vi "Parse Stored String (multibyte).vi"(1 "stored string":string caption="Gespeicherter String") -> (0 "parsed string":string caption="Untersuchter String")   [LabVIEW 2009]
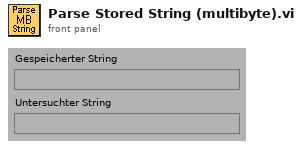
[diagram p1: front panel]
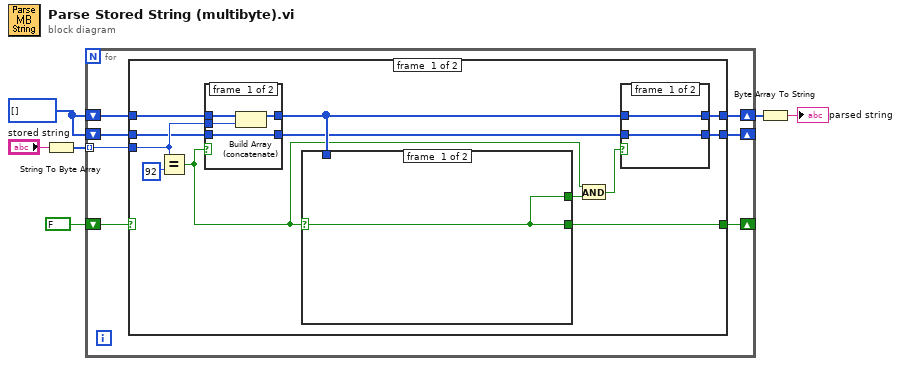
[diagram p0: block diagram]
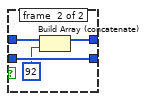
[diagram p2: hidden frame]
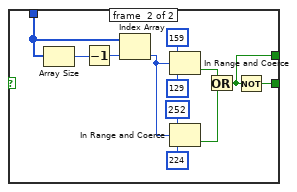
[diagram p3: hidden frame]
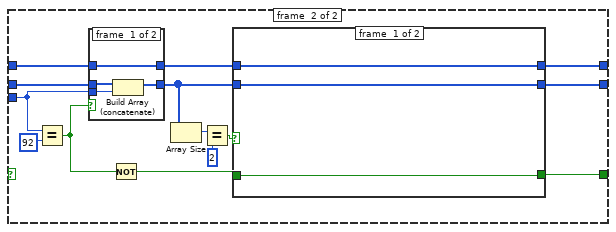
[diagram p5: hidden frame]
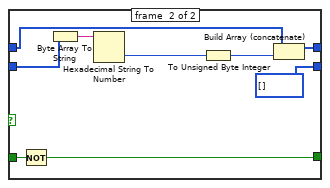
[diagram p6: hidden frame]
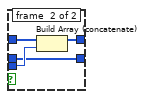
[diagram p7: hidden frame]
diagram:
  w1 = u8[] []
  n1 = String To Byte Array(string="stored string") -> (unsigned byte array=w3:u8[])
  n2 = for {
    tunnel: w3 -> [w9] mode=indexing
    shift-right: [w12] -> w4
    shift-left: w1 -> [w13]
    shift-right: [w10] -> _
    shift-left: FALSE -> [w11]
    shift-right: [w7] -> _
    shift-left: w1 -> [w8]
    n3 = case shown="False" w11 {
      tunnel: w13 -> [w24 w64]
      tunnel: [w17 w54] -> w12
      tunnel: [w21 w52] -> w10
      tunnel: w9 -> [w23 w51]
      tunnel: w8 -> [w22 w61]
      tunnel: [w16 w56] -> w7
      frame #0 {
        n4 = Equal?(x=w23, y=u8 92) -> (x = y?=w14:bool)
        n5 = case shown="False" w14 {
          tunnel: [w47 w50] -> w19
          tunnel: w24 -> [w48 w50]
          tunnel: w23 -> [w46 _]
          tunnel: [w45 w49] -> w18
          tunnel: w22 -> [w45 w49]
          frame #0 {
            n6 = Build Array (concatenate)(w48, w46) -> (w47:u8[])
          }
          frame #1 {
          }
        }
        n7 = case shown="False" w14 {
          selector: w14 -> [w32 _]
          tunnel: w19 -> [_ w42]
          tunnel: [w32 w34] -> w21
          tunnel: [w32 w33] -> w20
          frame #0 {
          }
          frame #1 {
            n8 = Array Size(array=w42) -> (size(s)=w44:i32)
            n9 = Decrement(x=w44) -> (x-1=w43:i32)
            n10 = Index Array(array=w42, index=w43) -> (element=w35:u8)
            n11 = In Range and Coerce(upper limit=u8 159, x=w35, lower limit=u8 129) -> (In Range?=w37:bool)  [unwired: 1 out]
            n12 = In Range and Coerce(upper limit=u8 252, x=w35, lower limit=u8 224) -> (In Range?=w36:bool)  [unwired: 1 out]
            n13 = Or(x=w37, y=w36) -> (x .or. y?=w33:bool)
            n14 = Not(x=w33) -> (.not. x?=w34:bool)
          }
        }
        n15 = And(x=w14, y=w20) -> (x .and. y?=w15:bool)
        n16 = case shown="True" w15 {
          tunnel: [w27 w30] -> w17
          tunnel: w19 -> [w27 w31]
          tunnel: [w26 w29] -> w16
          tunnel: w18 -> [w26 w29]
          frame #0 {
          }
          frame #1 {
            n17 = Build Array (concatenate)(w31, u8 92) -> (w30:u8[])
          }
        }
      }
      frame #1 {
        n18 = Equal?(x=w51, y=u8 92) -> (x = y?=w62:bool)
        n19 = case shown="False" w62 {
          tunnel: w64 -> [w80 w84]
          tunnel: [w80 w83] -> w55
          tunnel: w51 -> [w78 w82]
          tunnel: [w77 w81] -> w57
          tunnel: w61 -> [w79 w81]
          frame #0 {
            n20 = Build Array (concatenate)(w79, w78) -> (w77:u8[])
          }
          frame #1 {
            n21 = Build Array (concatenate)(w84, w82) -> (w83:u8[])
          }
        }
        n22 = Not(x=w62) -> (.not. x?=w53:bool)
        n23 = Array Size(array=w57) -> (size(s)=w60:i32)
        n24 = Equal?(x=w60, y=2) -> (x = y?=w58:bool)
        n25 = case shown="True" w58 {
          tunnel: [w67 u8[] []] -> w56
          tunnel: w57 -> [w67 w75]
          tunnel: [w66 w69] -> w54
          tunnel: w55 -> [w66 w71]
          tunnel: w53 -> [w65 w74]
          tunnel: [w65 w73] -> w52
          frame #0 {
          }
          frame #1 {
            n26 = Not(x=w74) -> (.not. x?=w73:bool)
            n27 = Byte Array To String(unsigned byte array=w75) -> (string=w72:string)
            n28 = Hexadecimal String To Number(string=w72) -> (number=w70:u32)  [unwired: 2 in, 1 out]
            n29 = To Unsigned Byte Integer(number=w70) -> (unsigned 8bit integer=w68:u8)
            n30 = Build Array (concatenate)(w71, w68) -> (w69:u8[])
          }
        }
      }
    }
  }
  n31 = Byte Array To String(unsigned byte array=w4) -> (string=→"parsed string":string)
